vi "Enable_VI_Checksums.vi"(8 "error in (no error)":errorcluster, 11 "AB_Build in":refnum<class "AB_Build.lvclass">) -> (0 "error out":errorcluster, 2 "VI checksums enabled?":bool, 3 "AB_Build out":refnum<class "AB_Build.lvclass">)   [LabVIEW 2020, in "AB_Build.lvclass"]
uses:
  <vilib>/AppBuilder/AB_Classes/Build/AB_Build.lvclass
  <vilib>/AppBuilder/AB_Classes/Build/AB_Build.lvclass/AB_Build.ctl
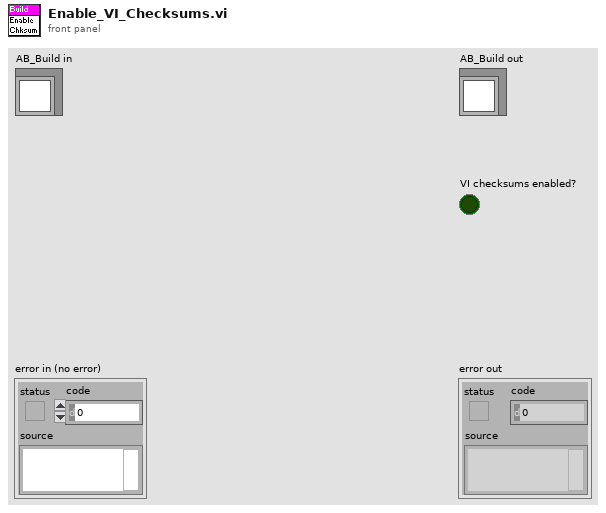
[diagram p1: front panel]
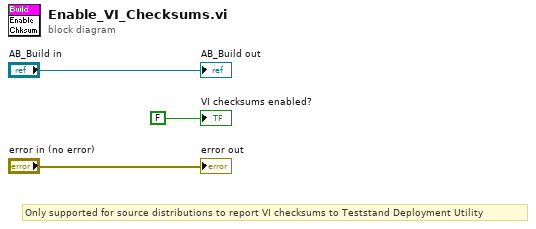
[diagram p0: block diagram]
diagram:
  # "Only supported for source distributions to report VI checksums to Teststand Deployment Utility"
  "error out" <- "error in (no error)"
  "AB_Build out" <- "AB_Build in"
  "VI checksums enabled?" <- FALSE ("VI checksums enabled?")
